vi "Agilent 34401 Read Multiple Measurements.vi"() -> ()   [LabVIEW 2011]
doc: "This example shows how to configure a measurement and take multiple readings."
uses:
  <vilib>/Utility/error.llb/DialogType.ctl
  <instrlib>/Agilent 34401/Public/Data/Read (Multiple Points).vi
  <instrlib>/Agilent 34401/Agilent 34401.lvlib
panel:
  in  "Maximum Time (10000 ms)":u32=10000
  in  "Function (0: DC Voltage)":u16(ring) items=["DC Voltage", "AC Voltage", "2 - Wire Resistance", "4 - Wire Resistance", "DC Current", "AC Current", "Frequency", "Period", "Continuity", "Diode Checking", "VDC:VDC Ratio", "Temperature", "Capacitance"]
  in  "Sample Count (10)":i32=10
  in  "Serial Configuration":T1={"Baud Rate"=9600, "Parity"=2, "Data Bits"=7} {"Data Bits" items=["7"=7, "8"=8]; "Parity" items=["None", "Odd", "Even"]; "Baud Rate" items=["300"=300, "600"=600, "1200"=1200, "2400"=2400, "4800"=4800, "9600"=9600, "19200"=19200]}
  out "Measurements":dbl[](array[numeric])
  in  "VISA resource name":refnum<visa-resource-name>
  # "(c) 2005-2008 National Instruments.  ALL RIGHTS RESERVED."
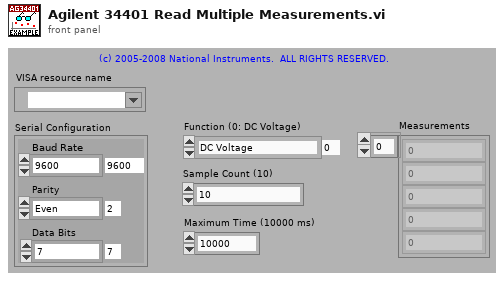
[diagram p1: front panel]
types:
  T1 = cluster{"Baud Rate":u32, "Parity":u16, "Data Bits":u16}
  T2 = typedef "DialogType.ctl" = u16
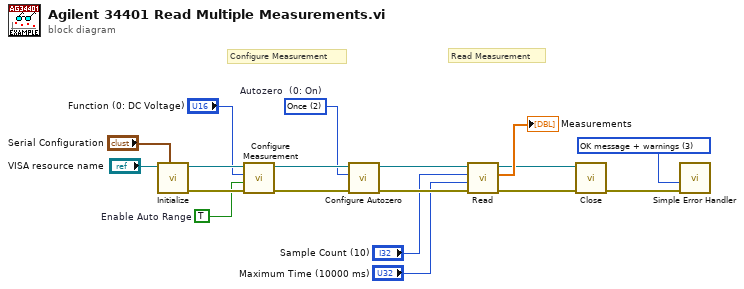
[diagram p0: block diagram]
diagram:
  w2 = T2 3 items=["no dialog", "OK message", "continue or stop message", "OK message + warnings", "continue/stop + warnings"] ("type of dialog (OK msg:1)")
  w9 = u16 2 items=["On", "Off", "Once"]  # Autozero  (0: On)
  w13 = TRUE  # Enable Auto Range
  # "Read Measurement"
  # "Configure Measurement"
  n1 = call <instrlib>:"Initialize.vi"("Serial Configuration"="Serial Configuration", "VISA resource name"="VISA resource name") -> ("error out"=w15:errorcluster, "VISA resource name out"=w16:refnum<visa-resource-name>)  [unwired: 8 in]
  n2 = call <instrlib>:"Configure Measurement.vi"("error in (no error)"=w15, "Enable Auto Range (T: Enable)"=w13, "Function (0: DC Voltage)"="Function (0: DC Voltage)", "VISA resource name"=w16) -> ("error out"=w11:errorcluster, "VISA resource name out"=w10:refnum<visa-resource-name>)  [unwired: 6 in]
  n3 = call <instrlib>:"Configure Autozero.vi"("error in (no error)"=w11, "Autozero  (0: On)"=w9, "VISA resource name"=w10) -> ("error out"=w5:errorcluster, "VISA resource name out"=w6:refnum<visa-resource-name>)  [unwired: 7 in]
  n4 = call-poly <instrlib>:"Read.vi"("error in (no error)"=w5, "Maximum Time (10000 ms)"="Maximum Time (10000 ms)", "Sample Count (1)"="Sample Count (10)", "VISA resource name"=w6) -> ("error out"=w7:errorcluster, "Measurements"=→"Measurements":dbl[], "VISA resource name out"=w8:refnum<visa-resource-name>)  [unwired: 5 in]
  n5 = call <instrlib>:"Close.vi"("error in (no error)"=w7, "VISA resource name"=w8) -> ("error out"=w18:errorcluster)  [unwired: 9 in]
  n6 = call <vilib>:"Simple Error Handler.vi"("type of dialog (OK msg:1)"=w2, "error in (no error)"=w18) -> ()  [unwired: 3 in, 5 out]
